vi "QCP_Set_I32.vi"(0 "QCP Data Block In":T1, 1 "QCP Name":string, 2 "Value In":i32) -> (7 "QCP Data Block Out":T1)   [LabVIEW 2016]
uses:
  <userlib>/836-Libraries/System/QCP_Support_Code/QCP_Data_Block.ctl
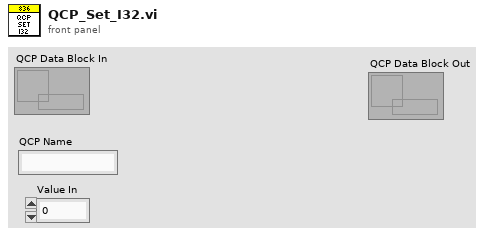
[diagram p1: front panel]
types:
  T1 = typedef "QCP_Data_Block.ctl" = refnum<data-value>
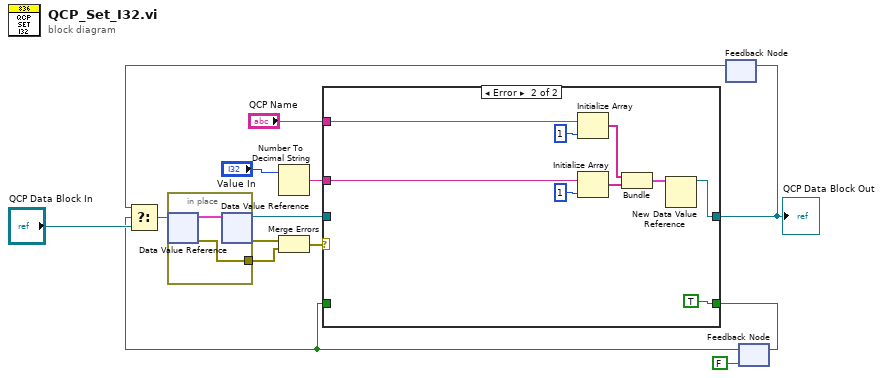
[diagram p0: block diagram]
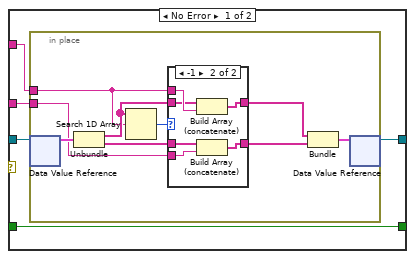
[diagram p2: hidden frame]
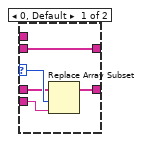
[diagram p3: hidden frame]
diagram:
  n1 = Number To Decimal String(number="Value In") -> (decimal integer string=w2:string)  [unwired: 1 in]
  n2 = feedback #1() -> (w3:T1)  [unwired: 1 in]
  n3 = feedback #2(FALSE) -> (w4:bool)
  n4 = Select(t=w3, s=w4, f="QCP Data Block In") -> (s? t:f=w5:T1)
  n5 = in-place {
    in-place-border: [w15] -> w13
    n6 = in-place-dvr #3(w5) -> (w16:cluster{string[], string[]}, w15:errorcluster)
    n7 = in-place-dvr #3(w16) -> (w11:T1, w14:errorcluster)
  }
  n8 = Merge Errors(w14, w13) -> (w12:errorcluster)
  n9 = case shown="Error" w12 {
    tunnel: [w21 w44] -> w9
    tunnel: w11 -> [w20 _]
    tunnel: "QCP Name" -> [w19 w50]
    tunnel: [w18 TRUE] -> w8
    tunnel: w4 -> [w18 _]
    tunnel: w2 -> [w17 w42]
    frame No Error {
      n10 = in-place {
        in-place-border: w19 -> [w23]
        in-place-border: w17 -> [w22]
        n11 = in-place-dvr #4(w20) -> (w30:cluster{string[], string[]})  [unwired: 1 out]
        n12 = Unbundle(w30) -> (w26:string[], w27:string[])
        n13 = Search 1D Array(1D array=w26, element=w23) -> (index of element=w28:i32)  [unwired: 1 out]
        n14 = case shown="-1" w28 {
          selector: w28 -> [w35 _]
          tunnel: w23 -> [_ w41]
          tunnel: [w32 w40] -> w25
          tunnel: w22 -> [w34 w39]
          tunnel: [w33 w38] -> w24
          tunnel: w27 -> [w31 w37]
          tunnel: w26 -> [w32 w36]
          frame 0, Default {
            n15 = Replace Array Subset(array=w31, new element=w34, index=w35) -> (w33:string[])
          }
          frame -1 {
            n16 = Build Array (concatenate)(w36, w41) -> (w40:string[])
            n17 = Build Array (concatenate)(w37, w39) -> (w38:string[])
          }
        }
        n18 = Bundle(w25, w24) -> (w29:cluster{string[], string[]})  [unwired: 1 in]
        n19 = in-place-dvr #4(w29) -> (w21:T1)  [unwired: 1 out]
      }
    }
    frame Error {
      n20 = Initialize Array(w50, 1 ("dimension size")) -> (w46:string[])
      n21 = Initialize Array(w42, 1 ("dimension size")) -> (w47:string[])
      n22 = Bundle(w46, w47) -> (w45:cluster{string[], string[]})  [unwired: 1 in]
      n23 = New Data Value Reference(data value=w45) -> (data value reference=w44:refnum<data-value>)  [unwired: 1 in, 1 out]
    }
  }
  "QCP Data Block Out" <- w9
  n24 = feedback-in #1(w9) -> ()
  n25 = feedback-in #2(w8) -> ()
